vi "Get Attribute BOOL.vi"(8 "error in":errorcluster, 10 "Attribute":string, 11 "IConfigurable in":refnum<class "IConfigurable.lvclass">) -> (0 "error out":errorcluster, 2 "Value":bool, 3 "IConfigurable out":refnum<class "IConfigurable.lvclass">)   [LabVIEW 2024, in "IConfigurable.lvclass"]
uses:
  IConfigurable.lvclass
  IConfiguration/IConfiguration.lvclass
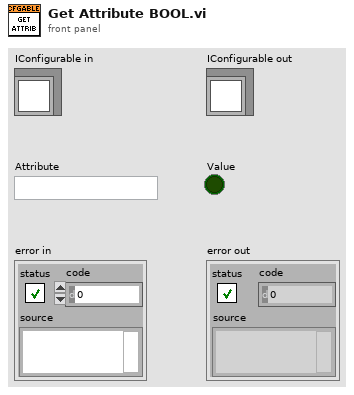
[diagram p1: front panel]
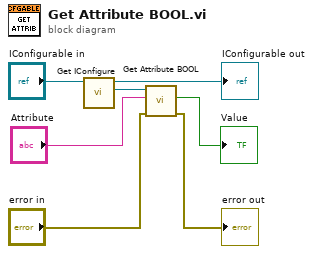
[diagram p0: block diagram]
diagram:
  n1 = call-dynamic "Get IConfigure.vi"("IConfigurable in"="IConfigurable in") -> ("IConfigure"=w5:refnum<class "IConfigure.lvclass">, "IConfigurable out"=→"IConfigurable out":refnum<class "IConfigurable.lvclass">)  [unwired: 8 in, 1 out]
  n2 = call-dynamic "Get Attribute BOOL.vi"("error in"="error in", "Attribute"="Attribute", "IConfiguration in"=w5) -> ("error out"=→"error out":errorcluster, "Value"=→"Value":bool)  [unwired: 6 in, 1 out]
